vi "Get_Files.vi"() -> ()   [LabVIEW 2010]
uses:
  File.lvclass
  LV_File.lvclass
panel:
  out "Selected External File Paths":path[](array[path])
  out "Selected VIs":string[](array[string])
  out "error out":errorcluster
  out "Open LV Files":T1(array[cluster])
  in  "error in (no error)":errorcluster
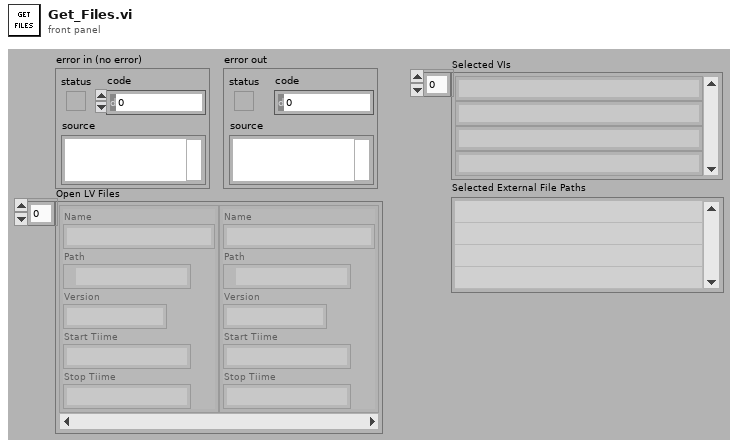
[diagram p1: front panel]
types:
  T1 = cluster{"Name":string, "Path":path, "Version":string, "Start Tiime":string, "Stop Tiime":string}[]
  T2 = cluster{"Name":string, "Path":path, "Version":string, "Start Tiime":string, "Stop Tiime":string}
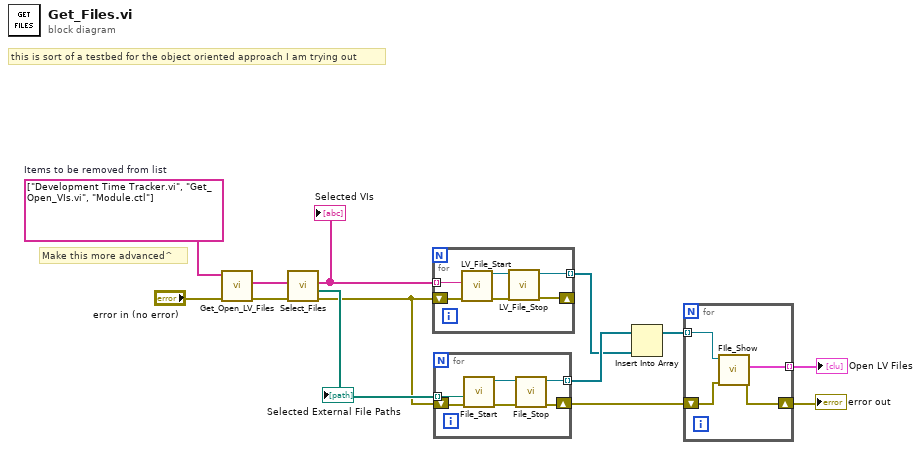
[diagram p0: block diagram]
diagram:
  w13 = string[] ["Development Time Tracker.vi", "Get_Open_VIs.vi", "Module.ctl"]  # Items to be removed from list
  # "this is sort of a testbed for the object oriented approach I am trying out"
  # "Make this more advanced^"
  n1 = call "Get_Open_LV_Files.vi"("error in (no error)"="error in (no error)", "Items to be ignored"=w13) -> ("error out"=w10:errorcluster, "Application:All VIs In Memory"=w11:string[])  [unwired: 8 in]
  n2 = call "Select_Files.vi"("error in"=w10, "Select Files"=w11) -> ("error out"=w7:errorcluster, "Selected External File Paths"=w8:path[], "Selected LV Files"=w9:string[])  [unwired: 7 in]
  "Selected VIs" <- w9
  "Selected External File Paths" <- w8
  n3 = for {
    shift-right: [w14] -> _
    shift-left: w7 -> [w17]
    tunnel: w9 -> [w16] mode=indexing
    tunnel: [w15] -> w1 mode=indexing
    n4 = call "LV_File_Start.vi"("error in"=w17, "VI Name"=w16) -> ("error out"=w19:errorcluster, "LV_File.lvclass (OUT)"=w18:refnum<class "LV_File.lvclass">)  [unwired: 8 in]
    n5 = call "LV_File_Stop.vi"("error in"=w19, "LV_File.lvclass (IN)"=w18) -> ("error out"=w14:errorcluster, "LV_File.lvclass (OUT)"=w15:refnum<class "LV_File.lvclass">)  [unwired: 8 in]
  }
  n6 = for {
    shift-right: [w21] -> w6
    shift-left: w7 -> [w20]
    tunnel: w8 -> [w25] mode=indexing
    tunnel: [w22] -> w2 mode=indexing
    n7 = call "File_Start.vi"("error in"=w20, "Path"=w25) -> ("error out"=w24:errorcluster, "File.lvclass (OUT)"=w23:refnum<class "File.lvclass">)  [unwired: 8 in]
    n8 = call "File_Stop.vi"("error in"=w24, "File.lvclass (IN)"=w23) -> ("error out"=w21:errorcluster, "File.lvclass (OUT)"=w22:refnum<class "File.lvclass">)  [unwired: 8 in]
  }
  n9 = Insert Into Array(array=w2, new element=w1) -> (w3:refnum<class "File.lvclass">[])  [unwired: 1 in]
  n10 = for {
    shift-right: [w28] -> w5
    shift-left: w6 -> [w29]
    tunnel: [w27] -> w4 mode=indexing
    tunnel: w3 -> [w26] mode=indexing
    n11 = call "FIle_Show.vi"("error in"=w29, "File.lvclass (IN)"=w26) -> ("error out"=w28:errorcluster, "File"=w27:T2)  [unwired: 7 in, 1 out]
  }
  "Open LV Files" <- w4
  "error out" <- w5
